vi "Parse Response JSON.vi"(8 "error in (no error)":errorcluster, 10 "Response JSON":string, 11 "RGetInputKindList in":refnum<class "RGetInputKindList.lvclass">) -> (0 "error out":errorcluster, 3 "RGetInputKindList out":refnum<class "RGetInputKindList.lvclass">)   [LabVIEW 2020, in "obs-websocket.lvlib" / "RGetInputKindList.lvclass"]
uses:
  RGetInputKindList.lvclass
  RGetInputKindList.lvclass/RGetInputKindList.ctl
  d43c8ed2-1994-48aa-af6c-d76456cc5fe2.vi
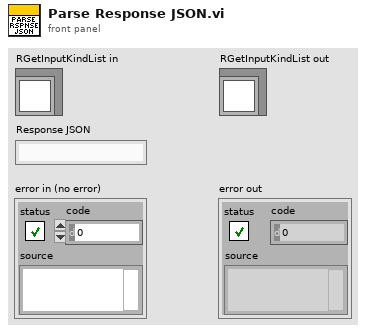
[diagram p1: front panel]
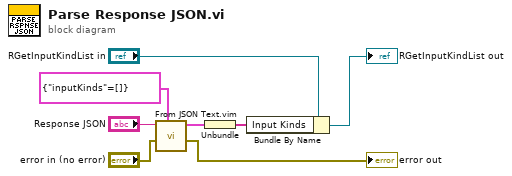
[diagram p0: block diagram]
diagram:
  n1 = call "From JSON Text.vim"("Data Type and Default Value"=cluster{"inputKinds":string[]} {"inputKinds"=[]}, "error in (no error)"="error in (no error)", "JSON"="Response JSON") -> ("error out"=→"error out":errorcluster, "Data out"=w2:cluster{"inputKinds":string[]})  [unwired: 7 in]
  n2 = Unbundle(w2) -> ("inputKinds"=w1:string[])
  n3 = Bundle By Name(cluster="RGetInputKindList in", "Input Kinds"=w1) -> (→"RGetInputKindList out":refnum<class "RGetInputKindList.lvclass">)
